vi "Teleop.vi"(10 "Match Info":T1={"Autonomous Elapsed Seconds"=0.0, "TeleOp Elapsed Seconds"=72.02, "Disabled Elapsed Seconds"=100.939, "Visited Autonomous"=FALSE, "Visited TeleOp"=TRUE, "Visited Disabled"=TRUE, "Autonomous Settings"={"Autonomous Style"=enum."Independent", "VI Refnum"=refnum}}, 11 "Call Context":T2=enum."Stop") -> ()   [LabVIEW 2017]
doc: "This VI is called for each enabled TeleOp packet received from the DS. It is typically used to read from joysticks and other inputs and update I/O or setpoints for timed control loops. It should complete and return within 20 milliseconds or risk missing DS packets."
uses:
  <vilib>/Rock Robotics/WPI/DriverStation/WPI_DriverStationDerivedRobotMode.ctl
  <vilib>/Rock Robotics/WPI/DriverStation/WPI_DriverStationMatch Info.ctl
  Configuration/JoystickData.ctl
  <vilib>/Rock Robotics/WPI/Utilities/WPI_GetSetVariantRefNum.vi
panel:
  # "Keep negative"
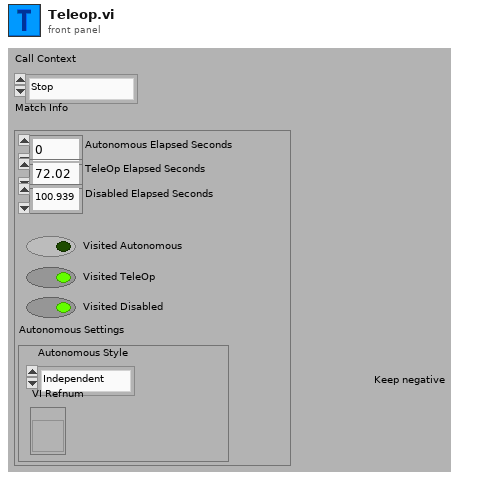
[diagram p1: front panel]
types:
  T1 = typedef "WPI_DriverStationMatch Info.ctl" = cluster{"Autonomous Elapsed Seconds":dbl, "TeleOp Elapsed Seconds":dbl, "Disabled Elapsed Seconds":dbl, "Visited Autonomous":bool, "Visited TeleOp":bool, "Visited Disabled":bool, "Autonomous Settings":cluster{"Autonomous Style":enum16{"Iterative", "Independent"}, "VI Refnum":refnum<vi>}}
  T2 = typedef "WPI_DriverStationDerivedRobotMode.ctl" = enum16{"Init", "Execute", "Stop"}
  T3 = typedef "JoystickData.ctl" = cluster{"DriveForward":dbl, "DriveTurn":dbl, "QuickTurn":bool}
  T4 = typedef "WPI_JoystickDevRef.ctl" = cluster{"Device":T5}
  T5 = typedef "WPI_JoystickDeviceEnum.ctl" = enum16{"USB 0", "USB 1", "USB 2", "USB 3", "USB 4", "USB 5"}
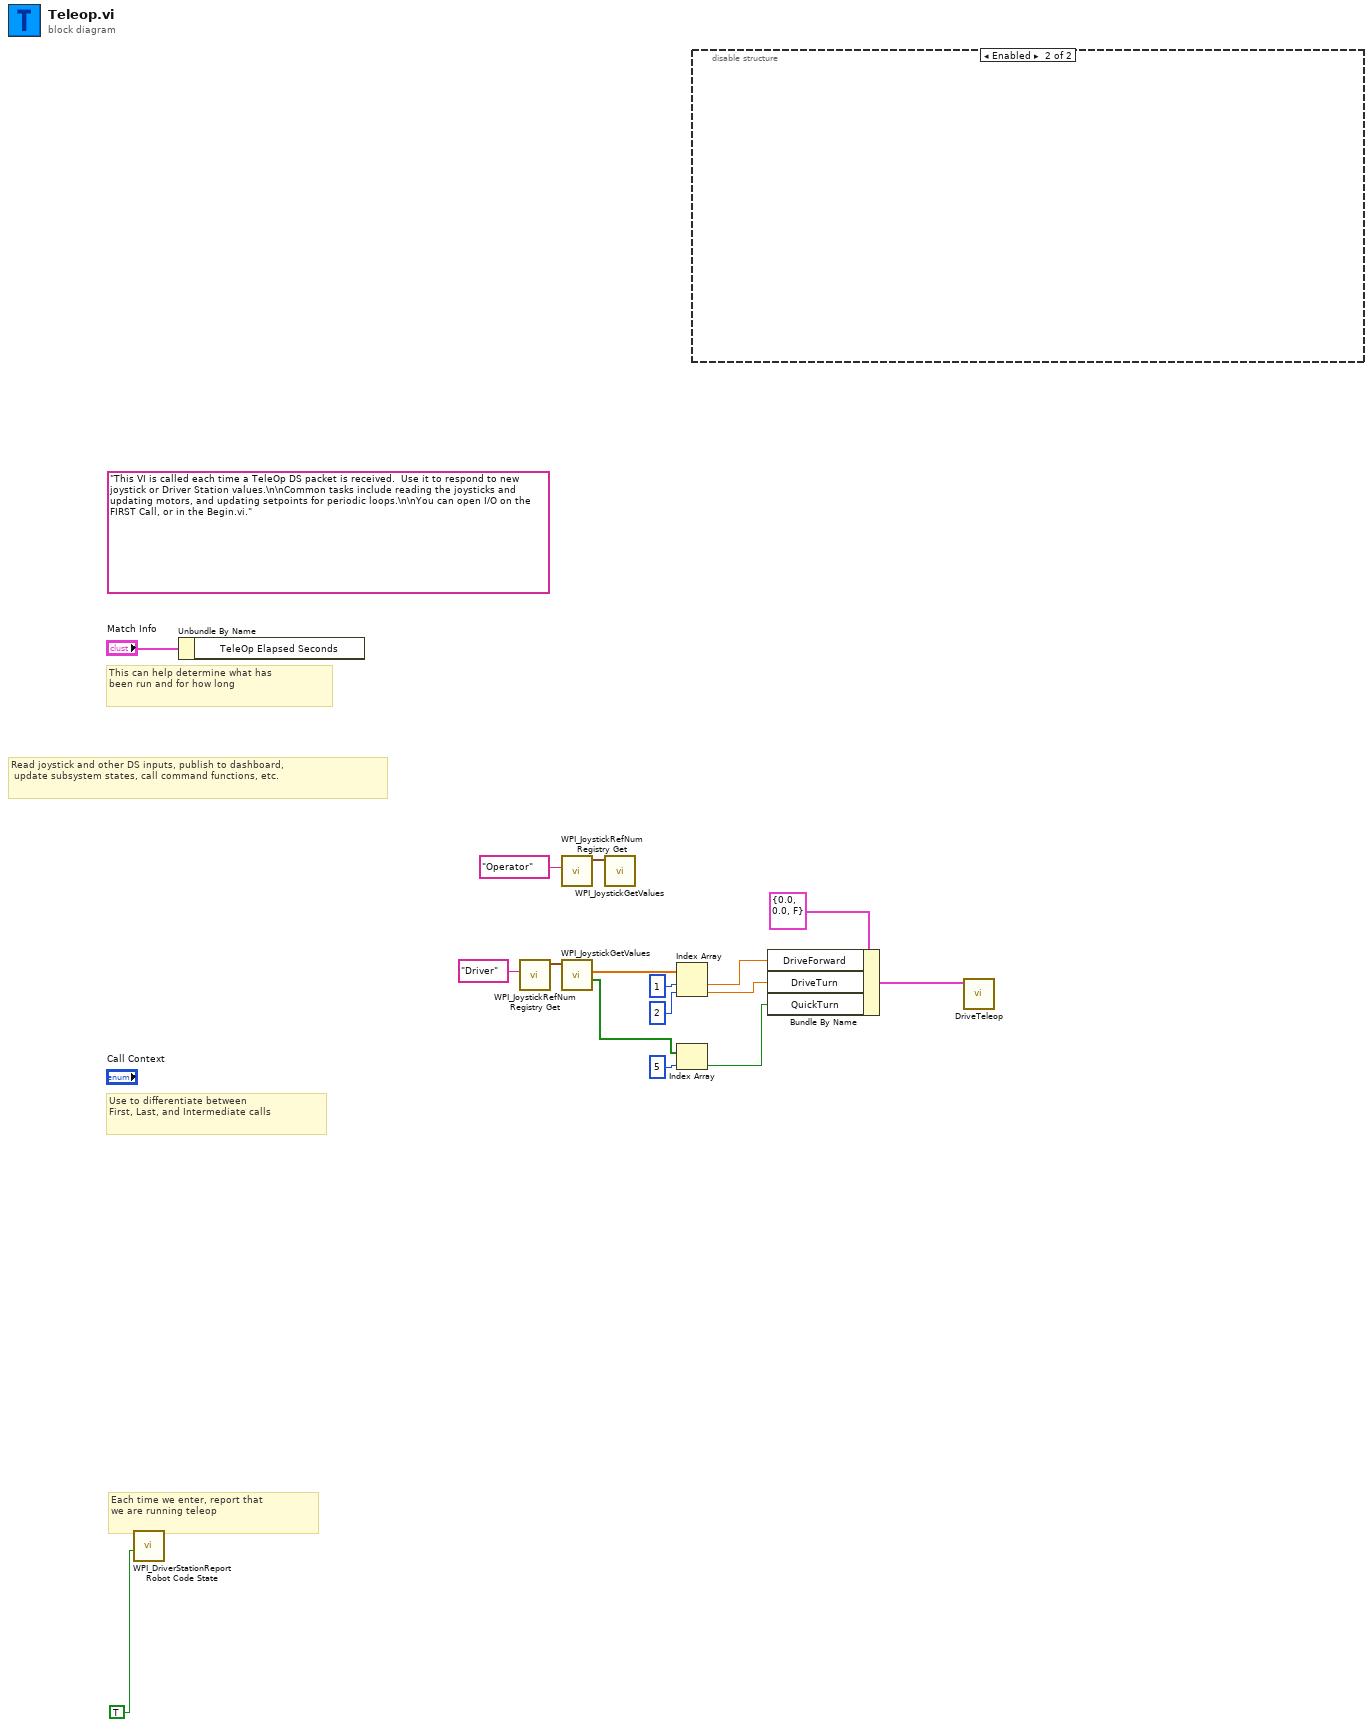
[diagram p0: block diagram]
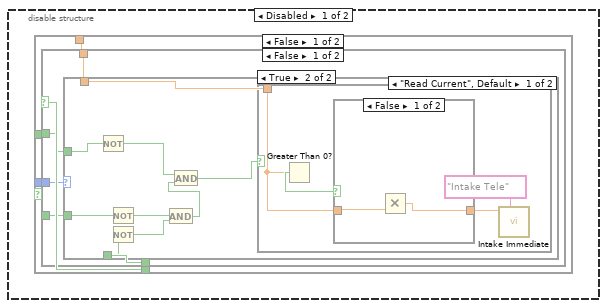
[diagram p2: hidden frame]
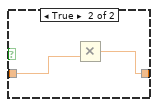
[diagram p4: hidden frame]
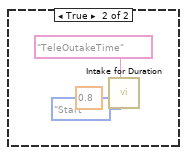
[diagram p6: hidden frame]
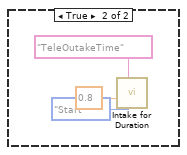
[diagram p7: hidden frame]
diagram:
  (unwired) "This VI is called each time a TeleOp DS packet is received.  Use it to respond to new joystick or Driver Station values.\n\nCommon tasks include reading the joysticks and updating motors, and updating setpoints for periodic loops.\n\nYou can open I/O on the FIRST Call, or in the Begin.vi."
  # "Read joystick and other DS inputs, publish to dashboard,\n update subsystem states, call command functions, etc."
  # "Each time we enter, report that\nwe are running teleop"
  # "Use to differentiate between\nFirst, Last, and Intermediate calls"
  # "This can help determine what has\nbeen run and for how long"
  n1 = call <vilib>:"WPI_DriverStationReport Robot Code State.vi"("TeleOp"=TRUE ("Autonomous")) -> ()  [unwired: 10 in, 1 out]
  n2 = Unbundle By Name("Match Info") -> ()  [unwired: 1 out]
  n3 = call <vilib>:"WPI_JoystickRefNum Registry Get.vi"("refnum name"="Driver") -> ("JoystickDevRef"=w12:T4)  [unwired: 1 in, 9 out]
  n4 = call <vilib>:"WPI_JoystickRefNum Registry Get.vi"("refnum name"="Operator") -> ("JoystickDevRef"=w14:T4)  [unwired: 1 in, 9 out]
  n5 = call <vilib>:"WPI_JoystickGetValues.vi"("JoystickDevRef"=w12) -> ("Buttons"=w6:bool[], "Axes"=w7:dbl[])  [unwired: 6 in, 3 out]
  n6 = call <vilib>:"WPI_JoystickGetValues.vi"("JoystickDevRef"=w14) -> ()  [unwired: 6 in, 5 out]
  n7 = Index Array(array=w7, index #1=1 ("index"), index #2=2 ("index")) -> (element #1=w3:dbl, element #2=w2:dbl)
  n8 = Index Array(array=w6, index=5) -> (element=w4:bool)
  n9 = disable-structure shown="Enabled" {
    frame Disabled {
      n10 = case shown="False" {
        selector: _ -> [_ _]
        tunnel: _ -> [w17 _]
        tunnel: _ -> [w20 _]
        tunnel: _ -> [w19 _]
        tunnel: _ -> [w18 _]
        frame False {
          n11 = case shown="False" w17 {
            tunnel: w20 -> [w25 _]
            tunnel: w19 -> [w24 _]
            tunnel: w18 -> [w23 _]
            tunnel: _ -> [w22 _]
            tunnel: w17 -> [w21 _]
            frame False {
              n12 = case shown="\"Read Current\", Default" w23 {
                tunnel: w25 -> [w34 _]
                tunnel: w24 -> [w33 _]
                tunnel: w22 -> [w31 _]
                tunnel: w21 -> [w30 _]
                frame "Read Current", Default {
                  n13 = Not(x=w33) -> (.not. x?=w32:bool)
                  n14 = Not(x=w31) -> (.not. x?=w29:bool)
                  n15 = Not(x=w30) -> (.not. x?=w28:bool)
                  n16 = And(x=w29, y=w28) -> (x .and. y?=w27:bool)
                  n17 = And(x=w32, y=w27) -> (x .and. y?=w26:bool)
                  n18 = case shown="True" w26 {
                    tunnel: w34 -> [_ w35]
                    frame False {
                    }
                    frame True {
                      n19 = Greater Than 0?(x=w35) -> (x > 0?=w37:bool)
                      n20 = case shown="False" w37 {
                        tunnel: w35 -> [w40 w42]
                        tunnel: [w39 w41] -> w36
                        frame False {
                          n21 = Multiply(y=w40) -> (x*y=w39:dbl)  [unwired: 1 in]
                        }
                        frame True {
                          n22 = Multiply(y=w42) -> (x*y=w41:dbl)  [unwired: 1 in]
                        }
                      }
                      n23 = call "Intake Immediate.vi"("Description"="Intake Tele", "Speed"=w36) -> ()  [unwired: 9 in, 1 out]
                    }
                  }
                }
                frame "Intake for Duration" {
                }
              }
            }
            frame True {
              n24 = call "Intake for Duration.vi"("Synchronization"=enum16{"Start", "Wait"}."Start", "Description"="TeleOutakeTime", "Duration (s)"=0.8) -> ()  [unwired: 8 in, 1 out]
            }
          }
        }
        frame True {
          n25 = call "Intake for Duration.vi"("Synchronization"=enum16{"Start", "Wait"}."Start", "Description"="TeleOutakeTime", "Duration (s)"=0.8) -> ()  [unwired: 8 in, 1 out]
        }
      }
    }
    frame Enabled {
    }
  }
  n26 = Bundle By Name(cluster=T3 {"DriveForward"=0.0, "DriveTurn"=0.0, "QuickTurn"=FALSE} ("JoystickData"), "DriveForward"=w3, "DriveTurn"=w2, "QuickTurn"=w4) -> (w1:T3)
  n27 = call "DriveTeleop.vi"("JoystickData"=w1) -> ()  [unwired: 11 in]
